vi "Write Outlet Thermistor Value.vi"(0 "Model IN":enum16{"Estar Centauro", "GFL"}(ring), 5 "Outlet Temperature":dbl, 11 "Error In":errorcluster) -> (15 "Error Out":errorcluster)   [LabVIEW 2016]
doc: "This VI generates a static analog voltage output representing the Outlet Temperature input."
uses:
  <vilib>/DAQmx/write.llb/DAQmx Write (Analog DBL 1Chan 1Samp).vi
  <vilib>/DAQmx/create/channels.llb/DAQmx Create Channel (AO-Voltage-Basic).vi
  <vilib>/DAQmx/miscellaneous.llb/DAQmx Fill In Error Info.vi
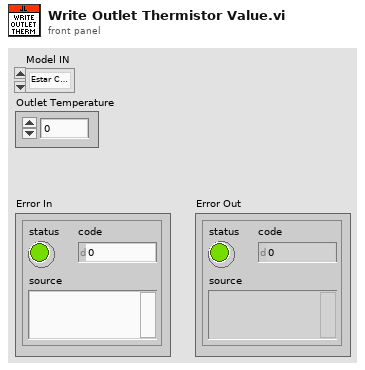
[diagram p1: front panel]
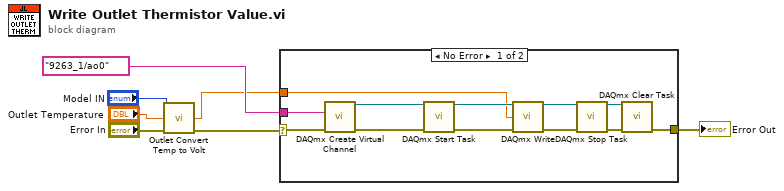
[diagram p0: block diagram]
diagram:
  n1 = call "Outlet Convert Temp to Volt.vi"("Model IN"="Model IN", "Outlet Temperature"="Outlet Temperature", "Error In"="Error In") -> ("Outlet Voltage"=w3:dbl, "Error Out"=w4:errorcluster)  [unwired: 11 in]
  n2 = case shown="No Error" w4 {
    selector: w4 -> [w11 w20]
    tunnel: tag "9263_1/ao0" ("Line") -> [w10 _]
    tunnel: w3 -> [w9 _]
    tunnel: [w8 w20] -> w6
    frame No Error {
      n3 = call-poly <vilib>:"DAQmx Create Virtual Channel.vi"("physical channels"=w10, "error in"=w11) -> ("task out"=w16:refnum<k21>, "error out"=w17:errorcluster)  [unwired: 12 in]
      n4 = call <vilib>:"DAQmx Start Task.vi"("task/channels in"=w16, "error in"=w17) -> ("task out"=w19:refnum<k21>, "error out"=w18:errorcluster)  [unwired: 12 in]
      n5 = call-poly <vilib>:"DAQmx Write.vi"("task/channels in"=w19, "data"=w9, "error in"=w18) -> ("task out"=w13:refnum<k21>, "error out"=w12:errorcluster)  [unwired: 10 in, 1 out]
      n6 = call <vilib>:"DAQmx Stop Task.vi"("task/channels in"=w13, "error in"=w12) -> ("task out"=w15:refnum<k21>, "error out"=w14:errorcluster)  [unwired: 12 in]
      n7 = call <vilib>:"DAQmx Clear Task.vi"("task in"=w15, "error in"=w14) -> ("error out"=w8:errorcluster)  [unwired: 13 in]
    }
    frame Error {
    }
  }
  "Error Out" <- w6
